vi "차선 인식(거리 클러스터, 기울기 클러스터.vi"() -> ()   [LabVIEW 2018]
uses:
  <vilib>/Math Plots/3D Math Plots/3D Scatter/3D Scatter XCtrl/3D Scatter.xctl
  <vilib>/Analysis/Matrix/Datatypes/RealMatrix.ctl
  <vilib>/Analysis/Matrix/Numeric/Conversions/Array To Matrix - RA.vi
  <vilib>/Analysis/Matrix/Numeric/Multiply/Multiply - RM,RM.vi
  <vilib>/Analysis/Matrix/Numeric/Conversions/Matrix To Array - RM.vi
  <vilib>/Math Plots/3D Math Plots/3D Scatter/3D Scatter Datatype/Public/Plot Helper (Vector).vi
  <vilib>/Math Plots/3D Math Plots/3D Scatter/3D Scatter Datatype/3D Scatter Datatype.lvclass
  <vilib>/Analysis/Matrix/NI_Matrix.lvlib
panel:
  out "차선 중앙 2":cluster{dbl[], dbl[]}(graph)
  out "차선 중앙":cluster{dbl[], dbl[]}(graph)
  out "왼쪽 차선":cluster{dbl[], dbl[]}(graph)
  out "오른쪽 차선":cluster{dbl[], dbl[]}(graph)
  out "반사율 꼬깔콘":cluster{dbl[], dbl[]}(graph)
  out "101이상 반사율":u8[](array[numeric])
  out "95~100반사율 배열":cluster{dbl, dbl, dbl, u8}[](array[cluster])
  out "반사율 xy(차선x)":cluster{dbl[], dbl[]}(graph)
  out "60미만 반사율":u8[](array[numeric])
  out "95이상 반사율":u8[](array[numeric])
  out "반사율 xy":cluster{dbl[], dbl[]}(graph)
  out "XZ 2":cluster{dbl[], dbl[]}(graph)
  out "클러스터링 후":cluster{dbl[], dbl[]}(graph)
  out "배열 5":cluster{dbl, dbl, dbl, i32}[](array[cluster])
  out "배열 2":u8[](array[numeric])
  out "XY 그래프":cluster{dbl[], dbl[]}(graph)
  out "azimuth 배열 사이즈":i32
  out "XZ":cluster{dbl[], dbl[]}(graph)
  out "YZ":cluster{dbl[], dbl[]}(graph)
  out "XY":cluster{dbl[], dbl[]}(graph)
  out "3D Scatter":refnum<class "3D Plot Datatype.lvclass">[](xcontrol)
  out "범위내의 X,Y,Z,반사율":cluster{dbl, dbl, dbl, u8}[](array[cluster])
  out "substring":string
  out "Array":string[](array[string])
  out "distance":dbl[](array[numeric])
  out "output array":u8[](array[numeric])
  in  "Boolean":bool
  out "xz":cluster{dbl[], dbl[]}(graph)
  out "yz":cluster{dbl[], dbl[]}(graph)
  out "XY Graph":cluster{dbl[], dbl[]}(graph)
  out "unsigned byte array":u8[][][](array[numeric])
  out "azimuth":dbl[](array[numeric])
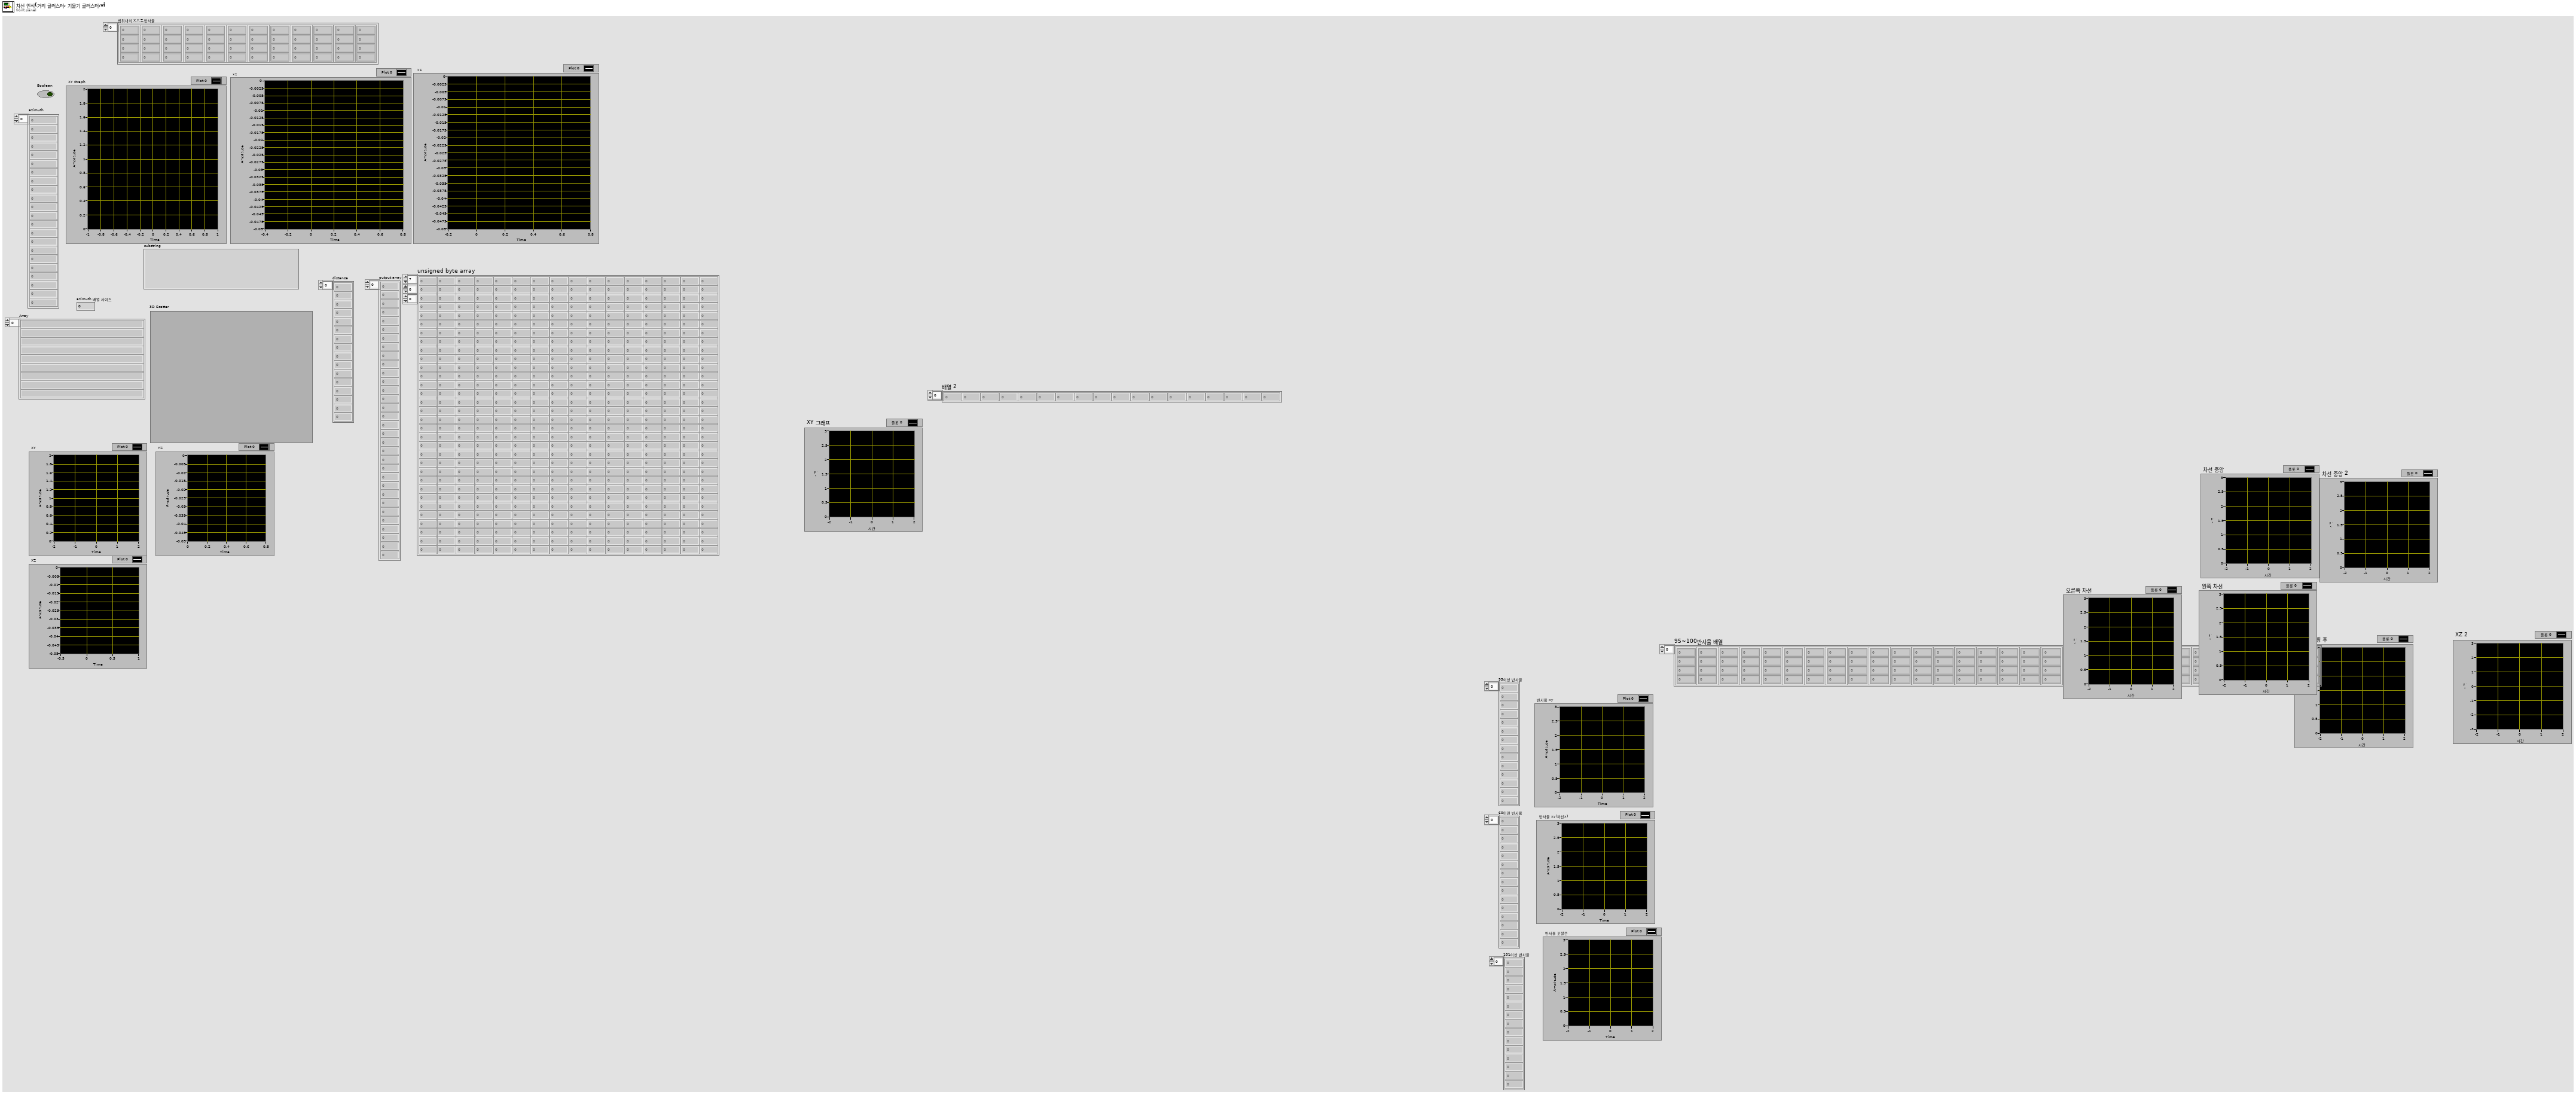
[diagram p1: front panel]
types:
  T1 = typedef "NI_Matrix.lvlib/RealMatrix.ctl" = dbl[][]
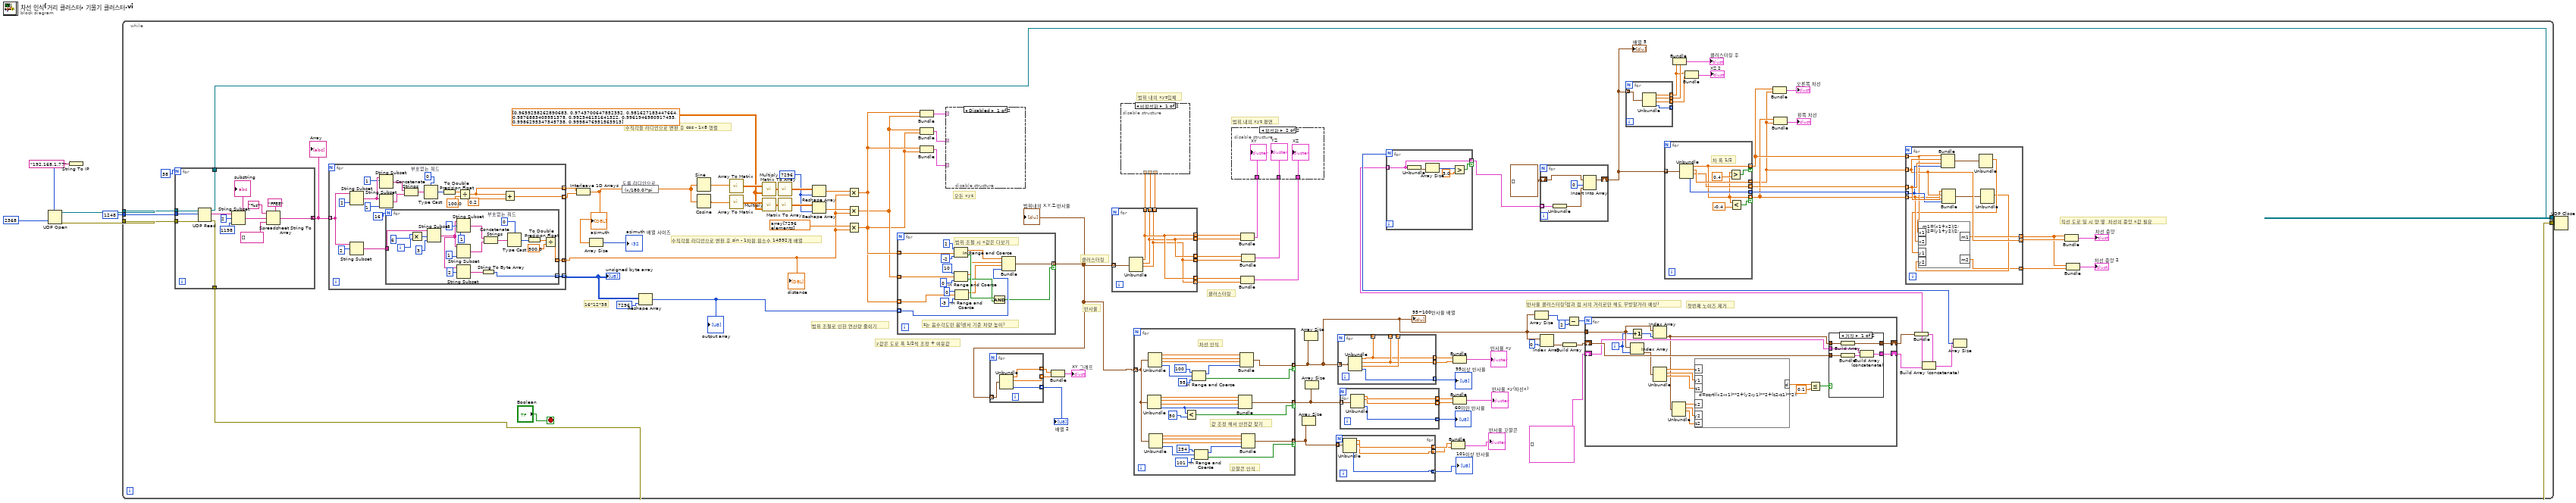
[diagram p0: block diagram]
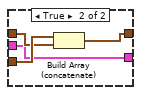
[diagram p2: hidden frame]
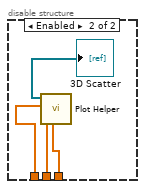
[diagram p4: hidden frame]
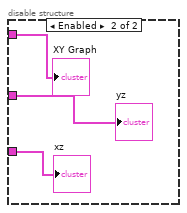
[diagram p5: hidden frame]
diagram:
  n1 = String To IP(1:"192.168.1.77") -> (0:w7:u32)
  n2 = UDP Open(7:w7, 11:2368) -> (port=w5:refnum<k16>, 0:w3:errorcluster)  [unwired: 3 in, 1 out]
  n3 = while {
    tunnel: w5 -> [w107]
    tunnel: 1248 -> [w106]
    tunnel: w3 -> [w105]
    tunnel: [w94] -> w2
    tunnel: [w77] -> w1
    stop <- "Boolean" stop-if-true
    w68 = 7296 ("차원 크기")
    w65 = T1 [[0.9659258262890683, 0.9743700647852352, 0.981627183447664, 0.9876883405951378, 0.992546151641322, 0.9961946980917455, 0.9986295347545738, 0.9998476951563913]] ("전치 행렬")
    # "첫번째 노이즈 제거"
    # "직선 도로 일 시 양 옆  차선의 중앙 x값 필요"
    # "y값은 도로 폭 1/2씩 조정 + 여윳값"
    # "반사율 클러스터링(점과 점 사의 거리로만 해도 무방할거라 예상)"
    # "범위 조절로 인한 연산량 줄이기"
    # "반사율"
    # "클러스터링"
    # "수직각을 라디언으로 변환 후 cos - 1x8 행렬"
    # "클러스터링"
    # "범위 내의 xyz 평면"
    # "범위 내의 xyz입체"
    # "모든 xyz"
    # "16*12*38"
    # "수직각을 라디언으로 변환 후 sin - 1차원 원소수 14592개 배열"
    n4 = for {
      N: 38 -> [_]
      tunnel: w107 -> [w298]
      tunnel: w106 -> [w297]
      tunnel: w105 -> [w296]
      tunnel: [w292] -> w94
      tunnel: [w287] -> w104 mode=concatenating
      tunnel: [w286] -> w77
      n5 = UDP Read(connection ID=w298, max size (548)=w297, 8:w296) -> (data out=w295:string, error out=w292:errorcluster, 3:w286:refnum<k16>)  [unwired: 1 in, 2 out]
      n6 = String Subset(string=w295, offset (0)=2, length (rest)=1198) -> (substring=w291:string)
      "substring" <- w291
      n7 = Spreadsheet String To Array(delimiter (Tab)="FFEE", format string="%s", spreadsheet string=w291, array type (2D Dbl)=string[] []) -> (array=w287:string[])
    }
    "Array" <- w104
    n8 = for {
      tunnel: w104 -> [w265] mode=indexing
      tunnel: [w252] -> w102 mode=indexing
      tunnel: [w251] -> w103 mode=indexing
      tunnel: [w248] -> w61 mode=concatenating
      tunnel: [w247] -> w101 mode=indexing
      w246 = u16 0  # 부호없는 워드
      n9 = String Subset(string=w265, offset (0)=2) -> (substring=w249:string)  [unwired: 1 in]
      n10 = String Subset(string=w265, length (rest)=2) -> (substring=w262:string)  [unwired: 1 in]
      n11 = String Subset(string=w262, offset (0)=1) -> (substring=w259:string)  [unwired: 1 in]
      n12 = String Subset(string=w262, length (rest)=1) -> (substring=w258:string)  [unwired: 1 in]
      n13 = for {
        N: 16 -> [_]
        tunnel: w249 -> [w285]
        tunnel: [w272] -> w248 mode=indexing
        tunnel: [w268] -> w247 mode=indexing
        i -> [w284]
        w266 = u16 0  # 부호없는 워드
        n14 = Multiply(x=6, y=w284) -> (x*y=w282:i32)
        n15 = String Subset(string=w285, offset (0)=w282, length (rest)=3) -> (substring=w271:string)
        n16 = String Subset(string=w271, offset (0)=2) -> (substring=w269:string)  [unwired: 1 in]
        n17 = String Subset(string=w271, offset (0)=1, length (rest)=1 ("length (rest)")) -> (substring=w278:string)
        n18 = String Subset(string=w271, length (rest)=1) -> (substring=w277:string)  [unwired: 1 in]
        n19 = String To Byte Array(string=w269) -> (unsigned byte array=w268:u8[])
        n20 = Concatenate Strings(w278, w277) -> (w276:string)
        n21 = Type Cast(type=w266, x=w276) -> (*(type *) &x=w275:u16)
        n22 = To Double Precision Float(number=w275) -> (double precision float=w274:dbl)
        n23 = Divide(x=w274, y=500.0) -> (x/y=w272:dbl)
      }
      n24 = Concatenate Strings(w259, w258) -> (w257:string)
      n25 = Type Cast(type=w246, x=w257) -> (*(type *) &x=w256:u16)
      n26 = To Double Precision Float(number=w256) -> (double precision float=w255:dbl)
      n27 = Divide(x=w255, y=100.0) -> (x/y=w251:dbl)
      n28 = Add(x=w251, y=0.2) -> (x+y=w252:dbl)
    }
    "unsigned byte array" <- w101
    "distance" <- w61
    n29 = Interleave 1D Arrays(w103, w102) -> (w79:dbl[])
    "azimuth" <- w79
    n30 = Array Size(array=w79) -> (size(s)=→"azimuth 배열 사이즈":i32)
    n31 = expression code="(x/180.0)*pi" "도를 라디안으로"(w79) -> (w90:dbl[])
    n32 = Reshape Array(w101, 7296 ("차원 크기")) -> (w99:u8[])
    "output array" <- w99
    n33 = Sine(x=w90) -> (sin(x)=w67:dbl[])
    n34 = Cosine(x=w90) -> (cos(x)=w66:dbl[])
    n35 = call-poly <vilib>:"Array To Matrix.vi"("Real 1D Array"=w67) -> ("Real Matrix (Column Vector)"=w74:T1)
    n36 = call-poly <vilib>:"Array To Matrix.vi"("Real 1D Array"=w66) -> ("Real Matrix (Column Vector)"=w73:T1)
    n37 = call-poly <vilib>:"Multiply.vi"("Real Matrix B"=w65, "Real Matrix A"=w74) -> ("A * B"=w72:T1)
    n38 = call-poly <vilib>:"Multiply.vi"("Real Matrix B"=w65, "Real Matrix A"=w73) -> ("A * B"=w71:T1)
    n39 = call-poly <vilib>:"Matrix To Array.vi"("Real Matrix"=w72) -> ("Real 2D Array"=w70:dbl[][])
    n40 = call-poly <vilib>:"Matrix To Array.vi"("Real Matrix"=w71) -> ("Real 2D Array"=w69:dbl[][])
    n41 = Reshape Array(w70, w68) -> (w64:dbl[])
    n42 = Reshape Array(w69, w68) -> (w63:dbl[])
    n43 = Multiply ("Multiply.vi")(x=w64, y=w61) -> (x*y=w93:dbl[])
    n44 = Multiply ("Multiply.vi")(x=w63, y=w61) -> (x*y=w92:dbl[])
    n45 = Multiply ("Multiply.vi")(x=dbl[] array[7296 elements] ("배열 2"), y=w61) -> (x*y=w91:dbl[])
    n46 = for {
      tunnel: w93 -> [w245] mode=indexing
      tunnel: w92 -> [w244] mode=indexing
      tunnel: w91 -> [w233] mode=indexing
      tunnel: w99 -> [w236] mode=indexing
      tunnel: [w235] -> w23 mode=indexing if=w234
      # "범위 조절 시 x값은 다보기"
      # "z는 음수각도만 봄(센서 기준 차량 높이)"
      n47 = In Range and Coerce(upper limit=2, x=w245, lower limit=-2) -> (coerced(x)=w238:dbl, In Range?=w240:bool)
      n48 = In Range and Coerce(upper limit=10, x=w244, lower limit=0) -> (coerced(x)=w237:dbl, In Range?=w239:bool)
      n49 = In Range and Coerce(upper limit=0, x=w233, lower limit=-3) -> (coerced(x)=w231:dbl)  [unwired: 1 out]
      n50 = Compound Arithmetic op=AND(w240, w239) -> (w234:bool)
      n51 = Bundle(w238, w237, w231, w236) -> (w235:cluster{dbl, dbl, dbl, u8})  [unwired: 1 in]
    }
    "범위내의 X,Y,Z,반사율" <- w23
    n52 = Bundle(w93, w92) -> (w98:cluster{dbl[], dbl[]})  [unwired: 1 in]
    n53 = Bundle(w92, w91) -> (w97:cluster{dbl[], dbl[]})  [unwired: 1 in]
    n54 = Bundle(w93, w91) -> (w96:cluster{dbl[], dbl[]})  [unwired: 1 in]
    n55 = disable-structure shown="Disabled" {
      disable-tunnel: w98 -> [_ w228]
      disable-tunnel: w97 -> [_ w227]
      disable-tunnel: w96 -> [_ w226]
      frame Disabled {
      }
      frame Enabled {
        "XY Graph" <- w228
        "yz" <- w227
        "xz" <- w226
      }
    }
    n56 = for {
      tunnel: w23 -> [w214] mode=indexing
      tunnel: [w213] -> w60 mode=indexing
      tunnel: [w212] -> w58 mode=indexing
      tunnel: [w211] -> w57 mode=indexing
      n57 = Unbundle(w214) -> (w213:dbl, w212:dbl, w211:u8)  [unwired: 1 out]
    }
    "배열 2" <- w57
    n58 = Bundle(w60, w58) -> (→"XY 그래프":cluster{dbl[], dbl[]})  [unwired: 1 in]
    n59 = for {
      tunnel: w23 -> [w225] mode=indexing
      tunnel: [w224] -> w76 mode=indexing
      tunnel: [w223] -> w75 mode=indexing
      tunnel: [w222] -> w89 mode=indexing
      tunnel: [w223] -> w88 mode=indexing
      tunnel: [w224] -> w87 mode=indexing
      tunnel: [w222] -> w86 mode=indexing
      tunnel: [w224] -> w85 mode=indexing
      tunnel: [w223] -> w84 mode=indexing
      tunnel: [w222] -> w83 mode=indexing
      n60 = Unbundle(w225) -> (w224:dbl, w223:dbl, w222:dbl)  [unwired: 1 out]
    }
    n61 = disable-structure shown="비활성화" {
      disable-tunnel: w85 -> [_ w220]
      disable-tunnel: w84 -> [_ w219]
      disable-tunnel: w83 -> [_ w218]
      frame Disabled {
      }
      frame Enabled {
        n62 = call-poly <vilib>:"Plot Helper.vi"("z vector"=w218, "y vector"=w219, "x vector"=w220) -> ("3D Plot lvclass Array out"=→"3D Scatter":refnum<class "3D Plot Datatype.lvclass">[])  [unwired: 3 in, 5 out]
      }
    }
    n63 = for {
      tunnel: w23 -> [w156] mode=indexing
      tunnel: [w164] -> w22 mode=indexing if=w151
      tunnel: [w160] -> w33 mode=indexing if=w157
      tunnel: [w152] -> w28 mode=indexing if=w142
      # "꼬깔콘 인식"
      # "차선 인식"
      # "값 조정 해서 안전값 찾기"
      n64 = Unbundle(w156) -> (w163:dbl, w162:dbl, w161:dbl, w159:u8)
      n65 = Unbundle(w156) -> (w167:dbl, w166:dbl, w165:dbl, w150:u8)
      n66 = Unbundle(w156) -> (w155:dbl, w154:dbl, w153:dbl, w146:u8)
      n67 = Less?(x=w159, y=50) -> (x < y?=w157:bool)
      n68 = In Range and Coerce(upper limit=100, x=w150, lower limit=95) -> (coerced(x)=w149:i32, In Range?=w151:bool)
      n69 = In Range and Coerce(upper limit=254, x=w146, lower limit=101) -> (coerced(x)=w143:i32, In Range?=w142:bool)
      n70 = Bundle(w163, w162, w161, w159) -> (w160:cluster{dbl, dbl, dbl, u8})  [unwired: 1 in]
      n71 = Bundle(w167, w166, w165, w149) -> (w164:cluster{dbl, dbl, dbl, i32})  [unwired: 1 in]
      n72 = Bundle(w155, w154, w153, w143) -> (w152:cluster{dbl, dbl, dbl, i32})  [unwired: 1 in]
    }
    "95~100반사율 배열" <- w22
    n73 = Bundle(w76, w75) -> (w82:cluster{dbl[], dbl[]})  [unwired: 1 in]
    n74 = Bundle(w87, w86) -> (w80:cluster{dbl[], dbl[]})  [unwired: 1 in]
    n75 = Bundle(w88, w89) -> (w81:cluster{dbl[], dbl[]})  [unwired: 1 in]
    n76 = disable-structure shown="활성화" {
      disable-tunnel: w82 -> [_ w215]
      disable-tunnel: w81 -> [_ w217]
      disable-tunnel: w80 -> [_ w216]
      frame Disabled {
      }
      frame Enabled {
        "XY" <- w215
        "YZ" <- w217
        "XZ" <- w216
      }
    }
    n77 = Array Size(array=w28) -> ()  [unwired: 1 out]
    n78 = Array Size(array=w22) -> ()  [unwired: 1 out]
    n79 = Array Size(array=w33) -> ()  [unwired: 1 out]
    n80 = for {
      tunnel: w28 -> [w132] mode=indexing
      tunnel: [w131] -> w27 mode=indexing
      tunnel: [w130] -> w26 mode=indexing
      tunnel: [w129] -> w25 mode=indexing
      n81 = Unbundle(w132) -> (w131:dbl, w130:dbl, w129:i32)  [unwired: 1 out]
    }
    "101이상 반사율" <- w25
    n82 = for {
      tunnel: [w137] -> w37 mode=indexing
      tunnel: [w138] -> w36 mode=indexing
      tunnel: [w141] -> w34 mode=indexing
      tunnel: w22 -> [w140] mode=indexing
      tunnel: [w139] -> _ mode=indexing
      tunnel: [w138] -> _ mode=indexing
      tunnel: [w137] -> _ mode=indexing
      n83 = Unbundle(w140) -> (w137:dbl, w138:dbl, w139:dbl, w141:i32)
    }
    "95이상 반사율" <- w34
    n84 = for {
      tunnel: w33 -> [w136] mode=indexing
      tunnel: [w135] -> w32 mode=indexing
      tunnel: [w134] -> w31 mode=indexing
      tunnel: [w133] -> w30 mode=indexing
      n85 = Unbundle(w136) -> (w134:dbl, w133:dbl, w135:u8)  [unwired: 1 out]
    }
    "60미만 반사율" <- w32
    n86 = Bundle(w27, w26) -> (→"반사율 꼬깔콘":cluster{dbl[], dbl[]})  [unwired: 1 in]
    n87 = Bundle(w37, w36) -> (→"반사율 xy":cluster{dbl[], dbl[]})  [unwired: 1 in]
    n88 = Bundle(w31, w30) -> (→"반사율 xy(차선x)":cluster{dbl[], dbl[]})  [unwired: 1 in]
    n89 = Array Size(array=w22) -> (size(s)=w56:i32)
    n90 = Index Array(array=w22, index=0 ("인덱스")) -> (element=w53:cluster{dbl, dbl, dbl, i32})
    n91 = Build Array(w53) -> (w54:cluster{dbl, dbl, dbl, i32}[])
    n92 = Subtract(x=w56, y=2) -> (x-y=w51:i32)
    n93 = for {
      N: w51 -> [_]
      tunnel: w22 -> [w199]
      shift-right: [w183] -> w41
      shift-left: w54 -> [w189]
      shift-right: [w187] -> w40
      shift-left: cluster{cluster{dbl, dbl, dbl, u8}[]}[] [] -> [w188]
      i -> [w184]
      n94 = Index Array(array=w199, index=w184) -> (element=w186:cluster{dbl, dbl, dbl, i32})
      n95 = Increment(x=w184) -> (x+1=w200:i32)
      n96 = Index Array(array=w199, index=w200) -> (element=w185:cluster{dbl, dbl, dbl, i32})
      n97 = Unbundle(w186) -> (w198:dbl, w197:dbl, w196:dbl)  [unwired: 1 out]
      n98 = Unbundle(w185) -> (w195:dbl, w194:dbl, w193:dbl)  [unwired: 1 out]
      n99 = formula code="d=sqrt((x2-x1)**2+(y2-y1)**2+(z2-z1)**2);"("x1"=w198, "y1"=w197, "z1"=w196, "x2"=w195, "y2"=w194, "z2"=w193) -> ("d"=w192:dbl)
      n100 = Less Or Equal?(x=w192, y=0.1) -> (x <= y?=w190:bool)
      n101 = case shown="거짓" w190 {
        tunnel: w189 -> [w206 w210]
        tunnel: w185 -> [w202 w209]
        tunnel: w188 -> [w205 w208]
        tunnel: [w203 w208] -> w187
        tunnel: [w201 w207] -> w183
        frame False {
          n102 = Build Array(w202) -> (w201:cluster{dbl, dbl, dbl, i32}[])
          n103 = Bundle(w206) -> (w204:cluster{cluster{dbl, dbl, dbl, i32}[]})  [unwired: 1 in]
          n104 = Build Array (concatenate)(w205, w204) -> (w203:cluster{cluster{dbl, dbl, dbl, i32}[]}[])
        }
        frame True {
          n105 = Build Array (concatenate)(w210, w209) -> (w207:cluster{dbl, dbl, dbl, i32}[])
        }
      }
    }
    n106 = Bundle(w41) -> (w42:cluster{cluster{dbl, dbl, dbl, i32}[]})  [unwired: 1 in]
    n107 = Build Array (concatenate)(w42, w40) -> (w38:cluster{cluster{dbl, dbl, dbl, i32}[]}[])
    n108 = Array Size(array=w38) -> (size(s)=w39:i32)
    n109 = for {
      N: w39 -> [_]
      tunnel: w38 -> [w178] mode=indexing
      tunnel: [w178] -> w48 mode=indexing if=w180
      n110 = Unbundle(w178) -> (w179:cluster{dbl, dbl, dbl, i32}[])
      n111 = Array Size(array=w179) -> (size(s)=w181:i32)
      n112 = Greater?(x=w181, y=3.0) -> (0:w180:bool)
    }
    n113 = for {
      shift-right: [w177] -> w21
      shift-left: cluster{dbl, dbl, dbl, i32}[] [] -> [w176]
      tunnel: w48 -> [w173] mode=indexing
      n114 = Unbundle(w173) -> (w175:cluster{dbl, dbl, dbl, i32}[])
      n115 = Insert Into Array(array=w176, index=0 ("인덱스"), new element=w175) -> (w177:cluster{dbl, dbl, dbl, i32}[])
    }
    "배열 5" <- w21
    n116 = for {
      tunnel: w21 -> [w172] mode=indexing
      tunnel: [w171] -> w44 mode=indexing
      tunnel: [w170] -> w47 mode=indexing
      tunnel: [w169] -> w45 mode=indexing
      tunnel: [w168] -> _ mode=indexing
      n117 = Unbundle(w172) -> (w171:dbl, w170:dbl, w169:dbl, w168:i32)
    }
    n118 = for {
      tunnel: w21 -> [w128] mode=indexing
      tunnel: [w121] -> w11 mode=indexing if=w127
      tunnel: [w126] -> w9 mode=indexing
      tunnel: [w125] -> w12 mode=indexing
      tunnel: [w124] -> w13 mode=indexing
      tunnel: [w121] -> w10 mode=indexing if=w123
      # "차 폭 1/2"
      n119 = Unbundle(w128) -> (w121:dbl, w126:dbl, w125:dbl, w124:i32)
      n120 = Greater?(x=w121, y=0.4) -> (0:w127:bool)
      n121 = Less?(x=w121, y=-0.4) -> (x < y?=w123:bool)
    }
    n122 = Bundle(w44, w47) -> (→"클러스터링 후":cluster{dbl[], dbl[]})  [unwired: 1 in]
    n123 = Bundle(w44, w45) -> (→"XZ 2":cluster{dbl[], dbl[]})  [unwired: 1 in]
    n124 = Bundle(w11, w9) -> (→"오른쪽 차선":cluster{dbl[], dbl[]})  [unwired: 1 in]
    n125 = Bundle(w10, w9) -> (→"왼쪽 차선":cluster{dbl[], dbl[]})  [unwired: 1 in]
    n126 = for {
      tunnel: w11 -> [w115] mode=indexing
      tunnel: w9 -> [w117] mode=indexing
      tunnel: w12 -> [w119] mode=indexing
      tunnel: w13 -> [w118] mode=indexing
      tunnel: w10 -> [w114] mode=indexing
      tunnel: [w117] -> w17 mode=indexing
      tunnel: [w116] -> w16 mode=indexing
      tunnel: [w109] -> w14 mode=indexing
      n127 = Bundle(w115, w117, w119, w118) -> (w112:cluster{dbl, dbl, dbl, i32})  [unwired: 1 in]
      n128 = Bundle(w114, w117, w119, w118) -> (w113:cluster{dbl, dbl, dbl, i32})  [unwired: 1 in]
      n129 = Unbundle(w112) -> (w111:dbl)  [unwired: 3 out]
      n130 = Unbundle(w113) -> (w110:dbl)  [unwired: 3 out]
      n131 = formula code="m1=(x1+x2)/2;\nm2=(y1+y2)/2;"("x1"=w115, "x2"=w114, "y1"=w111, "y2"=w110) -> ("m1"=w116:dbl, "m2"=w109:dbl)
    }
    n132 = Bundle(w16, w17) -> (→"차선 중앙":cluster{dbl[], dbl[]})  [unwired: 1 in]
    n133 = Bundle(w16, w14) -> (→"차선 중앙 2":cluster{dbl[], dbl[]})  [unwired: 1 in]
  }
  n134 = UDP Close(connection ID=w1, 8:w2) -> ()  [unwired: 2 out]
